vi "Main Remote.vi"() -> ()   [LabVIEW 2023]
uses:
  defs/Notification Definition.ctl
  defs/HTTP Queue Definition.ctl
  defs/Data.ctl
  <vilib>/Utility/sysdir.llb/System Directory Type.ctl
  <vilib>/userDefined/High Color/IMAQdx.ctl
panel:
  out "Photo Period [s]":u32
  out "Config ID":u32
  in  "Confirm Cameras":bool
  in  "RGB Camera Session":refnum<k21> caption="IMAQdx Session"
  in  "Stop":bool
  out "error out":errorcluster
  in  "Hyperspectral Camera Session":T1
  out "Photo Save Directory":path
  # "Config parameters get from BE"
  # "Cameras Initialization"
  # "Steps:\n - start VI\n - setup initialization parameters\n - confirm parameters"
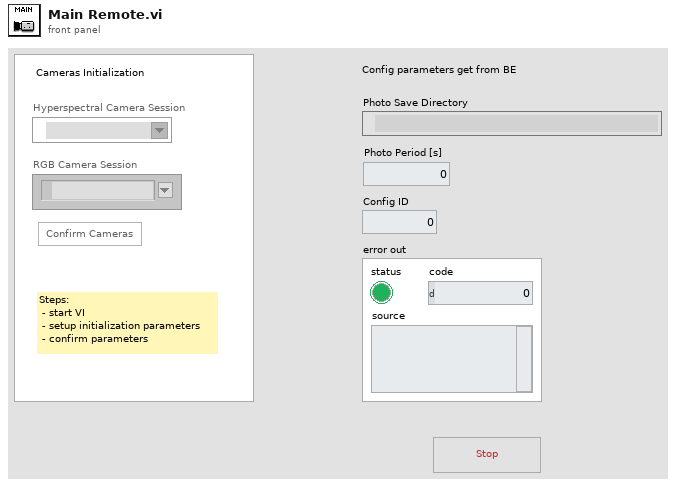
[diagram p1: front panel]
types:
  T1 = typedef "IMAQdx.ctl" = refnum<k21>
  T2 = typedef "System Directory Type.ctl" = i32
  T3 = typedef "Data.ctl" = cluster{"HTTP Queue":refnum<queue>, "Notifier":refnum<notifier>, "Photo Save Directory":path, "Photo Period (ms)":u32, "Cameras Enabled":cluster{"rgb_camera":bool, "hsi_camera":bool}, "Config ID":u32}
  T4 = typedef "HTTP Queue Definition.ctl" = cluster{"Message":string, "Photo Path":path}
  T5 = typedef "Notification Definition.ctl" = cluster{"Message":string}
  T6 = cluster{"id":i32, "interval_value":i32, "frequency":i32, "rgb_camera":bool, "hsi_camera":bool, "created_at":string}
  T7 = enum8{"Enabled", "Disabled", "Disabled and Grayed Out"}
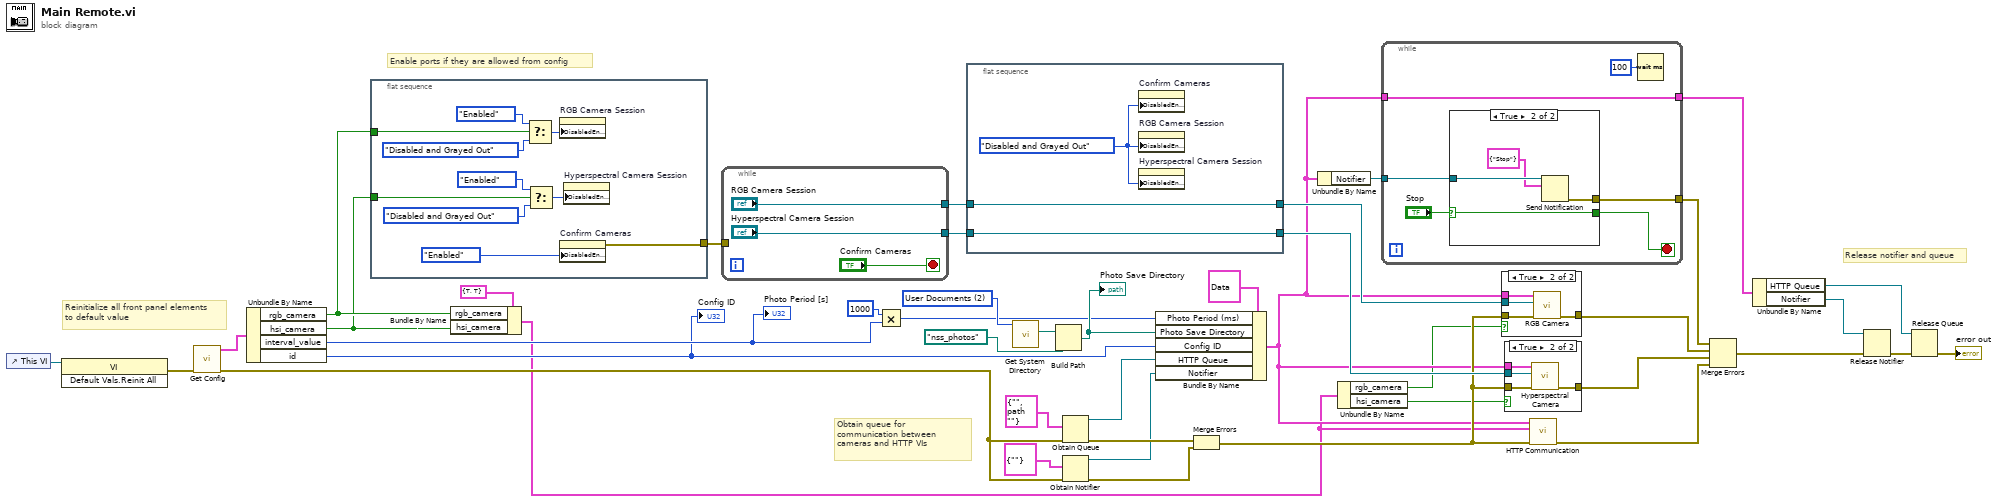
[diagram p0: block diagram]
diagram:
  w17 = T2 2 items=["User Home"=0, "User Desktop"=1, "User Documents"=2, "User Application Data"=3, "User Preferences"=4, "User Temporary"=5, "Public Documents"=6, "Public Application Data"=7, "Public Preferences"=8, "Public Cache"=13, "System Core Libraries"=9, "System Installed Libraries"=10, "Application Files"=11, "Boot Volume Root"=12] ("system directory type")
  # "Enable ports if they are allowed from config"
  # "Release notifier and queue"
  # "Obtain queue for communication between cameras and HTTP VIs"
  # "Reinitialize all front panel elements to default value"
  n1 = control-ref of="This VI"() -> (w29:refnum<vi>)
  n2 = invoke class="VI" method="Default Vals.Reinit All"(reference=w29) -> (error out=w34:errorcluster)  [unwired: 2 in, 2 out]
  n3 = call "Get Config.vi"("error in (no error)"=w34) -> ("error out"=w26:errorcluster, "Config"=w11:T6)  [unwired: 9 in]
  n4 = Unbundle By Name(w11) -> ("rgb_camera"=w8:bool, "hsi_camera"=w7:bool, "interval_value"=w10:i32, "id"=w2:i32)
  "Config ID" <- w2
  "Photo Period [s]" <- w10
  n5 = flat-sequence {
    tunnel: [w52] -> w28
    tunnel: w8 -> [w48]
    tunnel: w7 -> [w44]
    frame #0 {
      n6 = Select(t=T7."Enabled" ("Disabled"), s=w48, f=T7."Disabled and Grayed Out" ("Disabled")) -> (s? t:f=w49:T7)
      n7 = Select(t=T7."Enabled" ("Disabled"), s=w44, f=T7."Disabled and Grayed Out" ("Disabled")) -> (s? t:f=w45:T7)
      n8 = property on="RGB Camera Session" class="IMAQdx (strict)"("DisabledEnum"=w49) -> ()  [unwired: 2 in, 2 out]
      n9 = property on="Confirm Cameras" class="Bool"("DisabledEnum"=T7."Enabled" ("Disabled")) -> (error out=w52:errorcluster)  [unwired: 2 in, 1 out]
      n10 = property on="Hyperspectral Camera Session" class="IMAQdx (strict)"("DisabledEnum"=w45) -> ()  [unwired: 2 in, 2 out]
    }
  }
  n11 = Bundle By Name(cluster=cluster{"rgb_camera":bool, "hsi_camera":bool} {"rgb_camera"=TRUE, "hsi_camera"=TRUE}, "rgb_camera"=w8, "hsi_camera"=w7) -> (w1:cluster{"rgb_camera":bool, "hsi_camera":bool})
  n12 = while {
    tunnel: ["Hyperspectral Camera Session"] -> w32
    tunnel: ["RGB Camera Session"] -> w33
    tunnel: w28 -> [_]
    stop <- "Confirm Cameras" stop-if-true
  }
  n13 = Multiply(x=u32 1000, y=w10) -> (x*y=w12:u32)
  n14 = flat-sequence {
    tunnel: w33 -> [w57]
    tunnel: w32 -> [w58]
    tunnel: [w58] -> w31
    tunnel: [w57] -> w30
    frame #0 {
      w59 = T7."Disabled and Grayed Out" ("Disabled")
      n15 = property on="Confirm Cameras" class="Bool"("DisabledEnum"=w59) -> ()  [unwired: 2 in, 2 out]
      n16 = property on="RGB Camera Session" class="IMAQdx (strict)"("DisabledEnum"=w59) -> ()  [unwired: 2 in, 2 out]
      n17 = property on="Hyperspectral Camera Session" class="IMAQdx (strict)"("DisabledEnum"=w59) -> ()  [unwired: 2 in, 2 out]
    }
  }
  n18 = call <vilib>:"Get System Directory.vi"("system directory type"=w17) -> ("system directory"=w16:path)  [unwired: 10 in]
  n19 = Build Path(base path=w16, name or relative path=path "nss_photos") -> (appended path=w15:path)
  "Photo Save Directory" <- w15
  n20 = Obtain Queue(element data type=T4 {"Message"="", "Photo Path"=path ""}, error in (no error)=w26) -> (queue out=w3:refnum<queue>, error out=w25:errorcluster)  [unwired: 3 in, 1 out]
  n21 = Obtain Notifier(notification data type=T5 {"Message"=""} ("Event Handling Message"), error in (no error)=w26) -> (notifier out=w4:refnum<notifier>, error out=w24:errorcluster)  [unwired: 2 in, 1 out]
  n22 = Bundle By Name(cluster=T3 {"HTTP Queue"=refnum, "Notifier"=refnum, "Photo Save Directory"=path "", "Photo Period (ms)"=0, "Cameras Enabled"={"rgb_camera"=TRUE, "hsi_camera"=TRUE}, "Config ID"=0}, "Photo Period (ms)"=w12, "Photo Save Directory"=w15, "Config ID"=w2, "HTTP Queue"=w3, "Notifier"=w4) -> (w21:T3)
  n23 = Merge Errors(w25, w24) -> (w23:errorcluster)
  n24 = Unbundle By Name(w21) -> ("Notifier"=w22:refnum<notifier>)
  n25 = Unbundle By Name(w1) -> ("rgb_camera"=w6:bool, "hsi_camera"=w5:bool)
  n26 = while {
    tunnel: w22 -> [w65]
    tunnel: [w64] -> w39
    tunnel: w21 -> [w60]
    tunnel: [w60] -> w20
    stop <- w62 stop-if-true
    n27 = case shown="True" "Stop" {
      selector: "Stop" -> [_ w66]
      tunnel: w65 -> [_ w69]
      tunnel: [_ w68] -> w64
      tunnel: [_ w66] -> w62
      frame False {
      }
      frame True {
        n28 = Send Notification(notification=T5 {"Message"="Stop"}, notifier=w69) -> (error out=w68:errorcluster)  [unwired: 1 in, 1 out]
      }
    }
    n29 = Wait (ms)(milliseconds to wait=u32 100) -> ()  [unwired: 1 out]
  }
  n30 = case shown="True" w6 {
    tunnel: [w70 w74] -> w41
    tunnel: w30 -> [_ w73]
    tunnel: w23 -> [w70 w72]
    tunnel: w21 -> [_ w71]
    frame False {
    }
    frame True {
      n31 = call "RGB Camera.vi"("error in"=w72, "RGB Camera Session"=w73, "Data"=w71) -> ("error out"=w74:errorcluster)  [unwired: 8 in]
    }
  }
  n32 = case shown="True" w5 {
    tunnel: [w75 w79] -> w42
    tunnel: w31 -> [_ w78]
    tunnel: w23 -> [w75 w77]
    tunnel: w21 -> [_ w76]
    frame False {
    }
    frame True {
      n33 = call "Hyperspectral Camera.vi"("error in"=w77, "Hyperspectral Camera Session"=w78, "Data"=w76) -> ("error out"=w79:errorcluster)  [unwired: 8 in]
    }
  }
  n34 = call "HTTP Communication.vi"("error in"=w23, "Cameras Enabled"=w1, "Data"=w21) -> ("error out"=w37:errorcluster)  [unwired: 8 in]
  n35 = Merge Errors(w39, w41, w42, w37) -> (w40:errorcluster)
  n36 = Unbundle By Name(w20) -> ("HTTP Queue"=w18:refnum<queue>, "Notifier"=w19:refnum<notifier>)
  n37 = Release Notifier(notifier=w19, error in (no error)=w40) -> (error out=w36:errorcluster)  [unwired: 1 in, 2 out]
  n38 = Release Queue(queue=w18, error in (no error)=w36) -> (error out=→"error out":errorcluster)  [unwired: 1 in, 2 out]
